vi "StartMeas.vi"(8 "error in (no error)":errorcluster, 10 "Variant":variant, 11 "PacificPowerSource in":refnum<class "PacificPowerSource.lvclass">) -> (0 "error out":errorcluster, 3 "PacificPowerSource out":refnum<class "PacificPowerSource.lvclass">)   [LabVIEW 2018, in "AcPwrPlugins.lvlib" / "PacificPowerSource.lvclass"]
doc: "This VI starts the instrument measurement."
uses:
  PacificPowerSource.lvclass
panel:
  in  "Program Name":i32
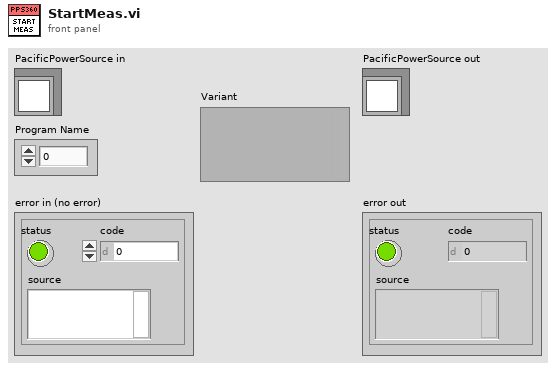
[diagram p1: front panel]
types:
  T1 = typedef "AcPwrPlugins.lvlib/PacificPowerSource.lvclass/Modules.ctl" = cluster{"Handle":string, "Connected":bool, "Clear Device (F)":bool, "btnIdQuery":bool, "btnReset":bool, "Program #":cluster{"Phase B (Degrees)":i32, "Waveform A (1: Sine)":i32, "Voltage Level (Va)":dbl, "Program Number (0)":i32, "Voltage Level (Vb) ":dbl, "Form (3: Three)":u16, "Coupling  (0: Direct)":u16, "Frequency (45Hz)":dbl, "Current Limit (40A)":dbl, "Phase C (Degrees)":i32, "Voltage Level (Vc)":dbl, "Waveform B (1: Sine)":i32, "Waveform C (1: Sine)":i32}[], "Impedance Parameters (off, 0.00)":cluster{"State":bool, "Impedance":dbl}, "Transient Execution (F)":bool, "OutputEnabled":bool, "Source Range":cluster{"Frequency Minimum (45 Hz)":dbl, "Frequency Maximum (1200 Hz)":dbl, "Voltage Maximum (V)":dbl, "Voltage Minimum (V)":dbl, "Range Control (0: Auto)":u16, "Initial Voltage (0V)":u16, "Frequency Range (600Hz)":u16}, "Port Type":enum16{"GPIB", "Serial"}}[]
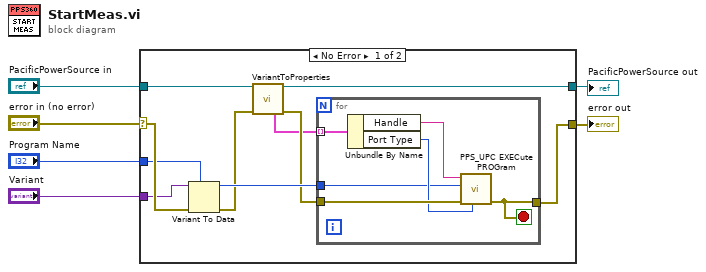
[diagram p0: block diagram]
diagram:
  n1 = case shown="No Error" "error in (no error)" {
    selector: "error in (no error)" -> [w15 w23]
    tunnel: "PacificPowerSource in" -> [w11 w24]
    tunnel: [w7 w24] -> w4
    tunnel: [w16 w23] -> w3
    tunnel: "Program Name" -> [w13 _]
    tunnel: "Variant" -> [w14 _]
    frame No Error {
      n2 = Variant To Data(error in=w15, type=w13, Variant=w14) -> (data=w12:i32, error out=w10:errorcluster)
      n3 = call "VariantToProperties.vi"("PacificPowerSource in"=w11, "error in (no error)"=w10) -> ("PacificPowerSource out"=w7:refnum<class "PacificPowerSource.lvclass">, "Modules"=w8:T1, "error out"=w9:errorcluster)  [unwired: 7 in, 4 out]
      n4 = for {
        tunnel: w8 -> [w22] mode=indexing
        tunnel: w9 -> [w20]
        tunnel: [w19] -> w16
        tunnel: w12 -> [w17]
        stop <- w19 stop-if-true
        n5 = Unbundle By Name(w22) -> ("Handle"=w21:string, "Port Type"=w18:enum16{"GPIB", "Serial"})
        n6 = call <instrlib>:"PPS_UPC EXECute PROGram.vi"("Port Type"=w18, "error in (no error)"=w20, "Program Name (1)"=w17, "VISA session"=w21) -> ("error out"=w19:errorcluster)  [unwired: 6 in, 1 out]
      }
    }
    frame Error {
    }
  }
  "error out" <- w3
  "PacificPowerSource out" <- w4
